vi "plotRobot.vi"(1 "L2":dbl, 4 "L1":dbl, 5 "y":dbl, 6 "x":dbl, 7 "y1":dbl, 8 "x1":dbl) -> (2 "XY Graph":cluster{dbl[], dbl[]}(graph))   [LabVIEW 2014]
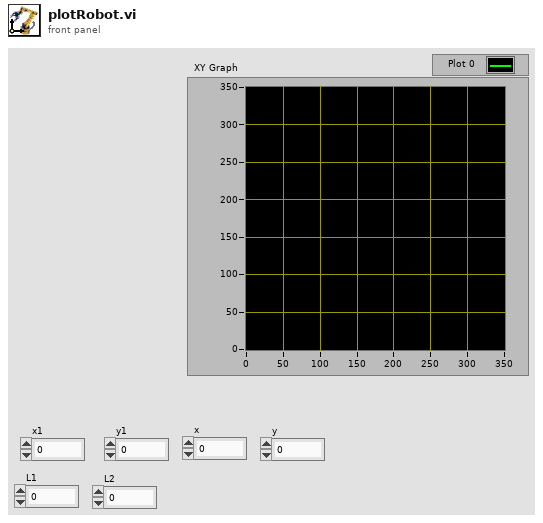
[diagram p1: front panel]
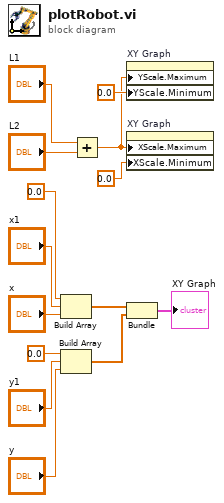
[diagram p0: block diagram]
diagram:
  n1 = Build Array "Build Array"(0.0 ("element"), "x1", "x") -> (w12:dbl[])
  n2 = Build Array "Build Array"(0.0 ("element"), "y1", "y") -> (w11:dbl[])
  n3 = Add(x="L1", y="L2") -> (x+y=w1:dbl)
  n4 = property on="XY Graph" class="XYGraph (strict)"("YScale.Maximum"=w1, "YScale.Minimum"=0.0 ("Y Scale.Range:Minimum")) -> ()  [unwired: 2 in, 2 out]
  n5 = property on="XY Graph" class="XYGraph (strict)"("XScale.Maximum"=w1, "XScale.Minimum"=0.0 ("X Scale.Range:Minimum")) -> ()  [unwired: 2 in, 2 out]
  n6 = Bundle "Bundle"(w12, w11) -> (→"XY Graph":cluster{dbl[], dbl[]})  [unwired: 1 in]
